vi "LowEnd-RT.vi"() -> ()   [LabVIEW 2016]
uses:
  <vilib>/rvi/interface/nirviOpenFPGA/nirviOpenFPGA.xnode
  <vilib>/rvi/interface/nirviReadWriteControl/nirviReadWriteControl.xnode
  LowEnd-FPGA.vi
  Controls/Glassman Control.ctl
  Controls/GP307 cluster.ctl
  Controls/Faraday cup states.ctl
  Controls/GV states.ctl
  Controls/Aperture states.ctl
  NiFpgaLv.dll
  <vilib>/Utility/error.llb/Error Cluster From Error Code.vi
  <vilib>/rvi/errors/niLvFpgaAdjustHostInterfaceError.vi
  <vilib>/NI_Real-Time Target Support.lvlib
  FPGA Bitfiles/PRIMEControl2017_FPGATarget2_LowEnd-FPGA_HC3RuQf6Dko.lvbitx
  <vilib>/FPGAPlugInAG/cRIO-9074/niLvFpga_Open_cRIO-9074.vi
panel:
  in  "Tab Control":T1(tab)
  out "LE Waist X+ Steerer V set":dbl
  out "LE Waist X+ Steerer HV Enable":bool
  out "LE Waist X- Steerer V set":dbl
  out "LE Waist X- Steerer HV Enable":bool
  out "LE Waist Y+ Steerer V set":dbl
  out "LE Waist Y+ Steerer HV Enable":bool
  out "LE Waist Y- Steerer V set":dbl
  out "LE Waist Y- Steerer HV Enable":bool
  out "LE Einzel V set":dbl
  out "LE Einzel HV Enable":bool
  out "LE Waist Y+ readback.V-monitor":fxp<+/-,16,5>
  out "LE Waist X+ readback.I-monitor":fxp<+/-,16,5>
  out "LE Waist X+ readback.V-monitor":fxp<+/-,16,5>
  out "LE Waist X- readback.I-monitor":fxp<+/-,16,5>
  out "LE Waist X- readback.V-monitor":fxp<+/-,16,5>
  out "LE Waist Y+ readback.I-monitor":fxp<+/-,16,5>
  out "LE Waist Y- readback.I-monitor":fxp<+/-,16,5>
  out "LE Waist Y- readback.V-monitor":fxp<+/-,16,5>
  out "LE Einzel readback.I-monitor":fxp<+/-,16,5>
  out "LE Einzel readback.V-monitor":fxp<+/-,16,5>
  out "Tank Entrance X+ Steerer HV Enable":bool
  out "Tank Entrance X+ Steerer V set":dbl
  out "Tank Entrance X- Steerer HV Enable":bool
  out "Tank Entrance X- Steerer V set":dbl
  out "Tank Entrance Y1+ Steerer HV Enable":bool
  out "Tank Entrance Y1+ Steerer V set":dbl
  out "Tank Entrance Y1- Steerer HV Enable":bool
  out "Tank Entrance Y1- Steerer V set":dbl
  out "Tank Entrance Y2+ Steerer HV Enable":bool
  out "Tank Entrance Y2+ Steerer V set":dbl
  out "Tank Entrance Y2- Steerer HV Enable":bool
  out "Tank Entrance Y2- Steerer V set":dbl
  out "Tank Entrance X+ readback.I-monitor":fxp<+/-,16,5>
  out "Tank Entrance X+ readback.V-monitor":fxp<+/-,16,5>
  out "Tank Entrance X- readback.I-monitor":fxp<+/-,16,5>
  out "Tank Entrance X- readback.V-monitor":fxp<+/-,16,5>
  out "Tank Entrance Y1+ readback.I-monitor":fxp<+/-,16,5>
  out "Tank Entrance Y1+ readback.V-monitor":fxp<+/-,16,5>
  out "Tank Entrance Y1- readback.I-monitor":fxp<+/-,16,5>
  out "Tank Entrance Y1- readback.V-monitor":fxp<+/-,16,5>
  out "Tank Entrance Y2+ readback.I-monitor":fxp<+/-,16,5>
  out "Tank Entrance Y2+ readback.V-monitor":fxp<+/-,16,5>
  out "Tank Entrance Y2- readback.I-monitor":fxp<+/-,16,5>
  out "Tank Entrance Y2- readback.V-monitor":fxp<+/-,16,5>
  out "LE Waist Vac Cluster":T2
  out "Tank Entrance Vac Cluster":T2
  out "LowEnd Waist Ion Gauge 1":u8[](array[numeric])
  out "LowEnd Waist Convectron 1":u8[](array[numeric])
  out "LowEnd Waist Ion Gauge 2":u8[](array[numeric])
  out "LowEnd Waist Convectron 2":u8[](array[numeric])
  out "LowEnd Waist Vac Interlock":bool
  out "Tank Entrance Vac Interlock":bool
  out "LowEnd Waist Vac Interlock bypass":bool
  out "Tank Entrance Vac Interlock bypass":bool
  out "Tank Entrance Ion Gauge 1":u8[](array[numeric])
  out "Tank Entrance Convectron 1":u8[](array[numeric])
  out "Tank Entrance Ion Gauge 2":u8[](array[numeric])
  out "Tank Entrance Convectron 2":u8[](array[numeric])
  out "Cryo Pump GV Position":T3
  out "Cryo Pump GV status":T4
  out "Beamline GV Position":T3
  out "Beamline GV status":T4
  out "Turbo GV Position":T3
  out "Turbo GV status":T4
  out "Tank Entrance FC Position":cluster{"IN sensor":bool, "OUT sensor":bool}
  out "Tank Entrance FC Status":T5
  out "LowEnd Waist FC Position":cluster{"IN sensor":bool, "OUT sensor":bool}
  out "LowEnd Waist FC Status":T5
  out "Bounce Mag Image  Aperture Position":cluster{"IN sensor":bool, "OUT sensor":bool}
  out "Bounce Mag Image  Aperture Position":T6
  out "Turbo GV actuator":bool
  out "Beamline GV actuator":bool
  out "Cryo Pump GV actuator":bool
  out "Tank Entrance FC actuator":bool
  out "LowEnd Waist FC actuator":bool
  out "Bounce Magnet Image Aperture actuator":bool
  out "Vac readback loop error":errorcluster
  out "HV control loop 2 error":errorcluster
  out "HV readback 2 loop error":errorcluster
  out "HV control 2 loop error":errorcluster
  out "Actuator-Sensor loop error":errorcluster
  out "HV readback 1 loop error":errorcluster
  out "GV Interlock loop error":errorcluster
  out "Error Handler":errorcluster
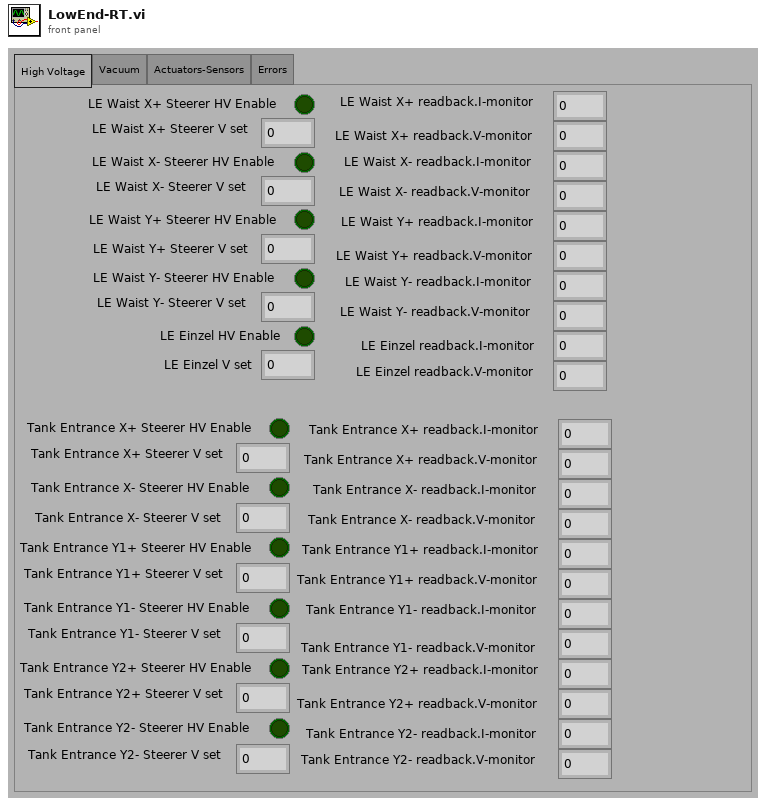
[diagram p1: front panel]
types:
  T1 = enum32{"High Voltage", "Vacuum", "Actuators-Sensors", "Errors"}
  T2 = cluster{"Ion gauge 1":string, "Convectron  Gauge 1 ":string, "Ion Gauge 2":string, "Convectrom Gauge 2":string}
  T3 = cluster{"OPEN sensor":bool, "Closed sensor":bool}
  T4 = typedef "GV states.ctl" = enum16{"status unclear", "closed", "open"}
  T5 = typedef "Faraday cup states.ctl" = enum16{"FC status unclear", "FC in", "FC out"}
  T6 = typedef "Aperture states.ctl" = enum16{"Aperture status unclear", "Aperture in", "Aperture out"}
  T7 = typedef "GP307 cluster.ctl" = cluster{"Ion gauge 1":string, "Convectron  Gauge 1 ":string, "Ion Gauge 2":string, "Convectrom Gauge 2":string}
  T8 = typedef "Glassman Control.ctl" = cluster{"V-program":fxp<+/-,16,5>, "HV Enable":bool}
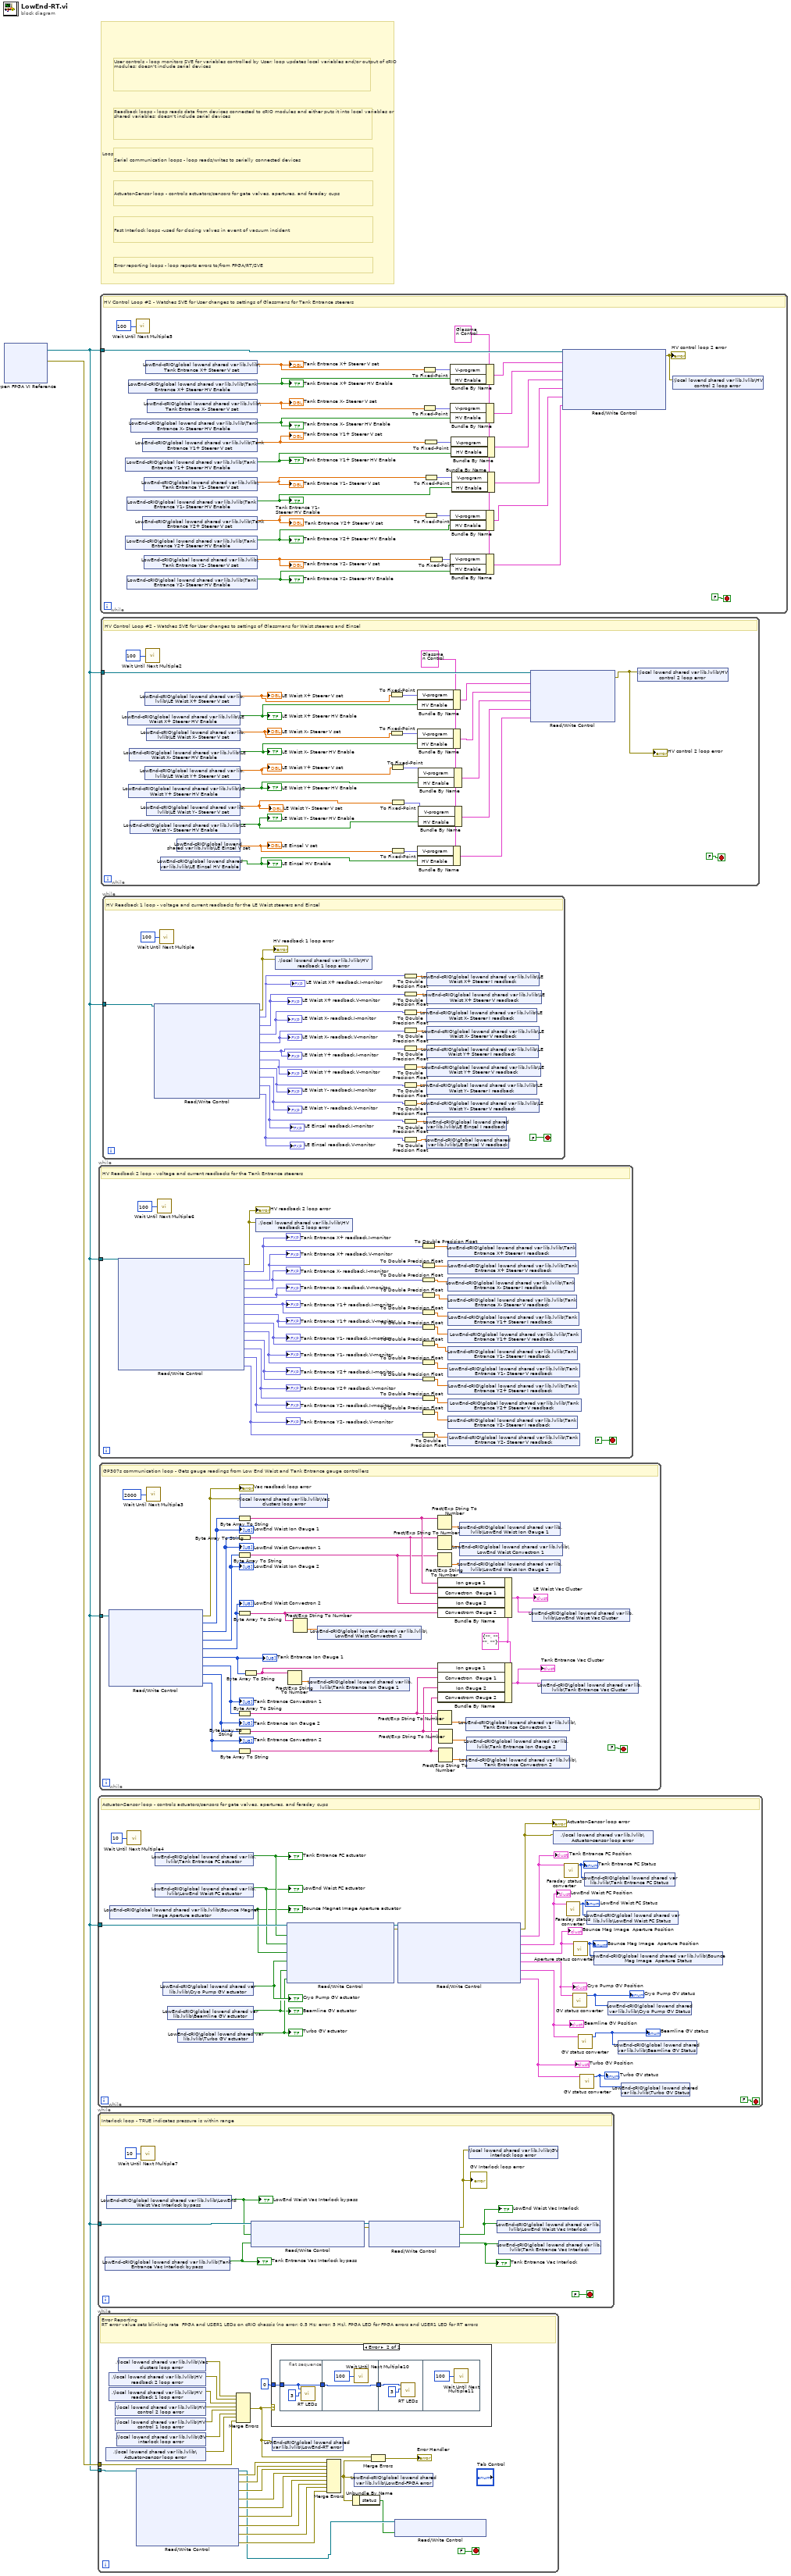
[diagram p0: block diagram]
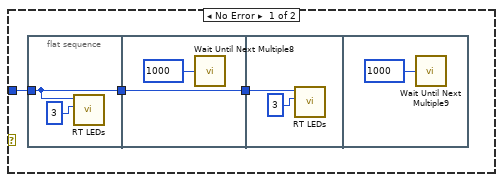
[diagram p2: hidden frame]
diagram:
  # "Actuator-Sensor loop - controls actuators/sensors for gate valves, apertures, and faraday cups"
  # "Fast Interlock loops -used for closing valves in event of vacuum incident"
  # "Error reporting loops - loop reports errors to/from FPGA/RT/SVE"
  # "Serial communication loops - loop reads/writes to serially connected devices"
  # "Readback loops - loop reads data from devices connected to cRIO modules and either puts it into local variables or shared variables; doesn't include serial devices"
  # "User controls - loop monitors SVE for variables controlled by User; loop updates local variables and/or output of cRIO modules; doesn't include serial devices"
  # "Loop legend - loops are color coded by responsibility"
  n1 = xnode "Open FPGA VI Reference"() -> ("FPGA VI Reference Out"=w1:refnum<k20>, "error out"=w2:errorcluster)  [unwired: 2 in]
  n2 = while {
    tunnel: w1 -> [w12]
    stop <- FALSE stop-if-true
    # "Interlock loop - TRUE indicates pressure is within range"
    n3 = shared-variable "LowEnd-cRIO\\global lowend shared var lib.lvlib\\Tank Entrance Vac Interlock bypass"() -> (w5:bool)  [unwired: 1 in, 1 out]
    "Tank Entrance Vac Interlock bypass" <- w5
    n4 = shared-variable "LowEnd-cRIO\\global lowend shared var lib.lvlib\\LowEnd Waist Vac Interlock bypass"() -> (w6:bool)  [unwired: 1 in, 1 out]
    "LowEnd Waist Vac Interlock bypass" <- w6
    n5 = call "Wait Until Next Multiple7"("Count(mSec)"=u32 10) -> ()  [unwired: 1 out]
    n6 = xnode "Read/Write Control"("FPGA VI Reference In"=w12, "LowEnd Waist Vac Interlock bypass"=w6, "Tank Entrance Vac Interlock bypass"=w5) -> ("FPGA VI Reference Out"=w11:refnum<k20>, "error out"=w10:errorcluster)  [unwired: 1 in]
    n7 = xnode "Read/Write Control"("FPGA VI Reference In"=w11, "error in"=w10) -> ("error out"=w9:errorcluster, "LowEnd Waist Vac Interlock"=w8:bool, "Tank Entrance Vac Interlock"=w7:bool)  [unwired: 1 out]
    "GV Interlock loop error" <- w9
    "LowEnd Waist Vac Interlock" <- w8
    "Tank Entrance Vac Interlock" <- w7
    n8 = shared-variable ".\\local lowend shared var lib.lvlib\\GV interlock loop error"(w9) -> ()  [unwired: 1 in, 1 out]
    n9 = shared-variable "LowEnd-cRIO\\global lowend shared var lib.lvlib\\LowEnd Waist Vac Interlock"(w8) -> ()  [unwired: 1 in, 1 out]
    n10 = shared-variable "LowEnd-cRIO\\global lowend shared var lib.lvlib\\Tank Entrance Vac Interlock"(w7) -> ()  [unwired: 1 in, 1 out]
  }
  n11 = while {
    tunnel: w1 -> [w36]
    tunnel: w2 -> [w16]
    stop <- FALSE stop-if-true
    # "Error Reporting\nRT error value sets blinking rate  FPGA and USER1 LEDs on cRIO chassis (no error: 0.5 Hz; error: 5 Hz). FPGA LED for FPGA errors and USER1 LED for RT errors"
    n12 = shared-variable ".\\local lowend shared var lib.lvlib\\Actuator-sensor loop error"() -> (w17:errorcluster)  [unwired: 1 in, 1 out]
    n13 = shared-variable ".\\local lowend shared var lib.lvlib\\HV readback 2 loop error"() -> (w22:errorcluster)  [unwired: 1 in, 1 out]
    n14 = shared-variable ".\\local lowend shared var lib.lvlib\\HV readback 1 loop error"() -> (w21:errorcluster)  [unwired: 1 in, 1 out]
    n15 = shared-variable ".\\local lowend shared var lib.lvlib\\HV control 2 loop error"() -> (w20:errorcluster)  [unwired: 1 in, 1 out]
    n16 = shared-variable ".\\local lowend shared var lib.lvlib\\HV control 1 loop error"() -> (w19:errorcluster)  [unwired: 1 in, 1 out]
    n17 = shared-variable ".\\local lowend shared var lib.lvlib\\GV interlock loop error"() -> (w18:errorcluster)  [unwired: 1 in, 1 out]
    n18 = shared-variable ".\\local lowend shared var lib.lvlib\\Vac clusters loop error"() -> (w23:errorcluster)  [unwired: 1 in, 1 out]
    n19 = xnode "Read/Write Control"("FPGA VI Reference In"=w36) -> ("FPGA VI Reference Out"=w25:refnum<k20>, "error out"=w26:errorcluster, "Low End Waist Vac Gauge error"=w27:errorcluster, "Tank Entrance Vac Gauge error"=w35:errorcluster, "GV Interlock loop error"=w34:errorcluster, "Actuator-sensor loop error"=w33:errorcluster, "HV control loop 1 error"=w32:errorcluster, "HV control loop 2 error"=w31:errorcluster, "HV readback loop #1 error"=w30:errorcluster, "HV readback loop #2 error"=w29:errorcluster)  [unwired: 1 in]
    n20 = Merge Errors(w23, w22, w21, w20, w19, w18, w17, w16) -> (w13:errorcluster)
    n21 = case shown="Error" w13 {
      tunnel: 0 -> [w40 w48]
      frame No Error {
        n22 = flat-sequence {
          tunnel: w40 -> [w41]
          tunnel: [w41] -> w38
          tunnel: [w43] -> w39
          tunnel: w38 -> [w43]
          tunnel: w39 -> [w45]
          frame #0 {
            n23 = call <vilib>:"RT LEDs.vi"("State"=3, "LED Num"=w41) -> ()  [unwired: 4 in, 2 out]
          }
          frame #1 {
            n24 = call "Wait Until Next Multiple8"("Count(mSec)"=u16 1000) -> ()  [unwired: 1 out]
          }
          frame #2 {
            n25 = call <vilib>:"RT LEDs.vi"("State"=3, "LED Num"=w45) -> ()  [unwired: 4 in, 2 out]
          }
          frame #3 {
            n26 = call "Wait Until Next Multiple9"("Count(mSec)"=u16 1000) -> ()  [unwired: 1 out]
          }
        }
      }
      frame Error {
        n27 = flat-sequence {
          tunnel: [w51] -> w50
          tunnel: w48 -> [w51]
          tunnel: w50 -> [w53]
          tunnel: [w53] -> w49
          tunnel: w49 -> [w55]
          frame #0 {
            n28 = call <vilib>:"RT LEDs.vi"("State"=3, "LED Num"=w51) -> ()  [unwired: 4 in, 2 out]
          }
          frame #1 {
            n29 = call "Wait Until Next Multiple10"("Count(mSec)"=u16 100) -> ()  [unwired: 1 out]
          }
          frame #2 {
            n30 = call <vilib>:"RT LEDs.vi"("State"=3, "LED Num"=w55) -> ()  [unwired: 4 in, 2 out]
          }
          frame #3 {
            n31 = call "Wait Until Next Multiple11"("Count(mSec)"=u16 100) -> ()  [unwired: 1 out]
          }
        }
      }
    }
    n32 = shared-variable "LowEnd-cRIO\\global lowend shared var lib.lvlib\\LowEnd-RT error"(w13) -> ()  [unwired: 1 in, 1 out]
    n33 = Merge Errors(w26, w27, w35, w34, w33, w32, w31, w30, w29) -> (w28:errorcluster)
    n34 = Unbundle By Name(w28) -> ("status"=w24:bool)
    n35 = shared-variable "LowEnd-cRIO\\global lowend shared var lib.lvlib\\LowEnd-FPGA error"(w28) -> ()  [unwired: 1 in, 1 out]
    n36 = Merge Errors(w13, w28) -> (→"Error Handler":errorcluster)
    n37 = xnode "Read/Write Control"("FPGA VI Reference In"=w25, "RT error"=w24) -> ()  [unwired: 1 in, 2 out]
  }
  n38 = while {
    tunnel: w1 -> [w81]
    stop <- FALSE stop-if-true
    # "Actuator-Sensor loop - controls actuators/sensors for gate valves, apertures, and faraday cups"
    n39 = shared-variable "LowEnd-cRIO\\global lowend shared var lib.lvlib\\Bounce Magnet Image Aperture actuator"() -> (w61:bool)  [unwired: 1 in, 1 out]
    "Bounce Magnet Image Aperture actuator" <- w61
    n40 = call "Wait Until Next Multiple4"("Count(mSec)"=u32 10) -> ()  [unwired: 1 out]
    n41 = shared-variable "LowEnd-cRIO\\global lowend shared var lib.lvlib\\LowEnd Waist FC actuator"() -> (w62:bool)  [unwired: 1 in, 1 out]
    "LowEnd Waist FC actuator" <- w62
    n42 = shared-variable "LowEnd-cRIO\\global lowend shared var lib.lvlib\\Tank Entrance FC actuator"() -> (w63:bool)  [unwired: 1 in, 1 out]
    "Tank Entrance FC actuator" <- w63
    n43 = shared-variable "LowEnd-cRIO\\global lowend shared var lib.lvlib\\Cryo Pump GV actuator"() -> (w60:bool)  [unwired: 1 in, 1 out]
    "Cryo Pump GV actuator" <- w60
    n44 = shared-variable "LowEnd-cRIO\\global lowend shared var lib.lvlib\\Beamline GV actuator"() -> (w58:bool)  [unwired: 1 in, 1 out]
    "Beamline GV actuator" <- w58
    n45 = shared-variable "LowEnd-cRIO\\global lowend shared var lib.lvlib\\Turbo GV actuator"() -> (w59:bool)  [unwired: 1 in, 1 out]
    "Turbo GV actuator" <- w59
    n46 = xnode "Read/Write Control"("FPGA VI Reference In"=w81, "Tank Entrance FC"=w63, "LowEnd Waist FC"=w62, "Bounce Magnet  Image Aperture"=w61, "Cryo Pump GV"=w60, "Beamline GV"=w58, "Turbo GV"=w59) -> ("FPGA VI Reference Out"=w79:refnum<k20>, "error out"=w77:errorcluster)  [unwired: 1 in]
    n47 = xnode "Read/Write Control"("FPGA VI Reference In"=w79, "error in"=w77) -> ("error out"=w64:errorcluster, "Tank Entrance FC Position"=w69:cluster{"IN sensor":bool, "OUT sensor":bool}, "LowEnd Waist FC Position"=w68:cluster{"IN sensor":bool, "OUT sensor":bool}, "Bounce Mag Image  Aperture Position"=w66:cluster{"IN sensor":bool, "OUT sensor":bool}, "Cryo Pump GV Position"=w75:T3, "Beamline GV Position"=w74:T3, "Turbo GV Position"=w73:T3)  [unwired: 1 out]
    "Cryo Pump GV Position" <- w75
    "Beamline GV Position" <- w74
    "Turbo GV Position" <- w73
    "Tank Entrance FC Position" <- w69
    "LowEnd Waist FC Position" <- w68
    "Bounce Mag Image  Aperture Position" <- w66
    "Actuator-Sensor loop error" <- w64
    n48 = shared-variable ".\\local lowend shared var lib.lvlib\\Actuator-sensor loop error"(w64) -> ()  [unwired: 1 in, 1 out]
    n49 = call "Faraday status converter.vi"("FC Position"=w69) -> ("FC Status"=w70:T5)  [unwired: 10 in]
    "Tank Entrance FC Status" <- w70
    n50 = call "Faraday status converter.vi"("FC Position"=w68) -> ("FC Status"=w67:T5)  [unwired: 10 in]
    "LowEnd Waist FC Status" <- w67
    n51 = call "GV status converter.vi"("Gate Valve"=w75) -> ("GV Status"=w71:T4)  [unwired: 10 in]
    "Cryo Pump GV status" <- w71
    n52 = call "Aperture status converter.vi"("Aperture Position"=w66) -> ("Aperture Status"=w65:T6)  [unwired: 10 in]
    "Bounce Mag Image  Aperture Position" <- w65
    n53 = call "GV status converter.vi"("Gate Valve"=w74) -> ("GV Status"=w76:T4)  [unwired: 10 in]
    "Beamline GV status" <- w76
    n54 = call "GV status converter.vi"("Gate Valve"=w73) -> ("GV Status"=w72:T4)  [unwired: 10 in]
    "Turbo GV status" <- w72
    n55 = shared-variable "LowEnd-cRIO\\global lowend shared var lib.lvlib\\Tank Entrance FC Status"(w70) -> ()  [unwired: 1 in, 1 out]
    n56 = shared-variable "LowEnd-cRIO\\global lowend shared var lib.lvlib\\LowEnd Waist FC Status"(w67) -> ()  [unwired: 1 in, 1 out]
    n57 = shared-variable "LowEnd-cRIO\\global lowend shared var lib.lvlib\\Bounce Mag Image  Aperture Status"(w65) -> ()  [unwired: 1 in, 1 out]
    n58 = shared-variable "LowEnd-cRIO\\global lowend shared var lib.lvlib\\Cryo Pump GV Status"(w71) -> ()  [unwired: 1 in, 1 out]
    n59 = shared-variable "LowEnd-cRIO\\global lowend shared var lib.lvlib\\Beamline GV Status"(w76) -> ()  [unwired: 1 in, 1 out]
    n60 = shared-variable "LowEnd-cRIO\\global lowend shared var lib.lvlib\\Turbo GV Status"(w72) -> ()  [unwired: 1 in, 1 out]
  }
  n61 = while {
    tunnel: w1 -> [w109]
    stop <- FALSE stop-if-true
    # "HV Readback 2 loop - voltage and current readbacks for the Tank Entrance steerers"
    n62 = xnode "Read/Write Control"("FPGA VI Reference In"=w109) -> ("error out"=w108:errorcluster, "Tank Entrance X+ readback.I-monitor"=w107:fxp<+/-,16,5>, "Tank Entrance X+ readback.V-monitor"=w106:fxp<+/-,16,5>, "Tank Entrance X- readback.I-monitor"=w105:fxp<+/-,16,5>, "Tank Entrance X- readback.V-monitor"=w104:fxp<+/-,16,5>, "Tank Entrance Y1+ readback.I-monitor"=w103:fxp<+/-,16,5>, "Tank Entrance Y1+ readback.V-monitor"=w102:fxp<+/-,16,5>, "Tank Entrance Y1- readback.I-monitor"=w101:fxp<+/-,16,5>, "Tank Entrance Y1- readback.V-monitor"=w100:fxp<+/-,16,5>, "Tank Entrance Y2+ readback.I-monitor"=w99:fxp<+/-,16,5>, "Tank Entrance Y2+ readback.V-monitor"=w98:fxp<+/-,16,5>, "Tank Entrance Y2- readback.I-monitor"=w97:fxp<+/-,16,5>, "Tank Entrance Y2- readback.V-monitor"=w96:fxp<+/-,16,5>)  [unwired: 1 in, 1 out]
    "HV readback 2 loop error" <- w108
    "Tank Entrance X+ readback.I-monitor" <- w107
    "Tank Entrance X+ readback.V-monitor" <- w106
    "Tank Entrance X- readback.I-monitor" <- w105
    "Tank Entrance X- readback.V-monitor" <- w104
    "Tank Entrance Y1+ readback.I-monitor" <- w103
    "Tank Entrance Y1+ readback.V-monitor" <- w102
    "Tank Entrance Y1- readback.I-monitor" <- w101
    "Tank Entrance Y1- readback.V-monitor" <- w100
    "Tank Entrance Y2+ readback.I-monitor" <- w99
    "Tank Entrance Y2+ readback.V-monitor" <- w98
    "Tank Entrance Y2- readback.I-monitor" <- w97
    "Tank Entrance Y2- readback.V-monitor" <- w96
    n63 = call "Wait Until Next Multiple6"("Count(mSec)"=u32 100) -> ()  [unwired: 1 out]
    n64 = shared-variable ".\\local lowend shared var lib.lvlib\\HV readback 2 loop error"(w108) -> ()  [unwired: 1 in, 1 out]
    n65 = To Double Precision Float(number=w107) -> (double precision float=w94:dbl)
    n66 = To Double Precision Float(number=w106) -> (double precision float=w93:dbl)
    n67 = To Double Precision Float(number=w105) -> (double precision float=w92:dbl)
    n68 = To Double Precision Float(number=w104) -> (double precision float=w91:dbl)
    n69 = To Double Precision Float(number=w103) -> (double precision float=w90:dbl)
    n70 = To Double Precision Float(number=w102) -> (double precision float=w89:dbl)
    n71 = To Double Precision Float(number=w101) -> (double precision float=w88:dbl)
    n72 = To Double Precision Float(number=w100) -> (double precision float=w87:dbl)
    n73 = To Double Precision Float(number=w99) -> (double precision float=w86:dbl)
    n74 = To Double Precision Float(number=w98) -> (double precision float=w85:dbl)
    n75 = To Double Precision Float(number=w97) -> (double precision float=w84:dbl)
    n76 = To Double Precision Float(number=w96) -> (double precision float=w83:dbl)
    n77 = shared-variable "LowEnd-cRIO\\global lowend shared var lib.lvlib\\Tank Entrance X+ Steerer I readback"(w94) -> ()  [unwired: 1 in, 1 out]
    n78 = shared-variable "LowEnd-cRIO\\global lowend shared var lib.lvlib\\Tank Entrance X+ Steerer V readback"(w93) -> ()  [unwired: 1 in, 1 out]
    n79 = shared-variable "LowEnd-cRIO\\global lowend shared var lib.lvlib\\Tank Entrance X- Steerer I readback"(w92) -> ()  [unwired: 1 in, 1 out]
    n80 = shared-variable "LowEnd-cRIO\\global lowend shared var lib.lvlib\\Tank Entrance X- Steerer V readback"(w91) -> ()  [unwired: 1 in, 1 out]
    n81 = shared-variable "LowEnd-cRIO\\global lowend shared var lib.lvlib\\Tank Entrance Y1+ Steerer I readback"(w90) -> ()  [unwired: 1 in, 1 out]
    n82 = shared-variable "LowEnd-cRIO\\global lowend shared var lib.lvlib\\Tank Entrance Y1+ Steerer V readback"(w89) -> ()  [unwired: 1 in, 1 out]
    n83 = shared-variable "LowEnd-cRIO\\global lowend shared var lib.lvlib\\Tank Entrance Y1- Steerer I readback"(w88) -> ()  [unwired: 1 in, 1 out]
    n84 = shared-variable "LowEnd-cRIO\\global lowend shared var lib.lvlib\\Tank Entrance Y1- Steerer V readback"(w87) -> ()  [unwired: 1 in, 1 out]
    n85 = shared-variable "LowEnd-cRIO\\global lowend shared var lib.lvlib\\Tank Entrance Y2+ Steerer I readback"(w86) -> ()  [unwired: 1 in, 1 out]
    n86 = shared-variable "LowEnd-cRIO\\global lowend shared var lib.lvlib\\Tank Entrance Y2+ Steerer V readback"(w85) -> ()  [unwired: 1 in, 1 out]
    n87 = shared-variable "LowEnd-cRIO\\global lowend shared var lib.lvlib\\Tank Entrance Y2- Steerer I readback"(w84) -> ()  [unwired: 1 in, 1 out]
    n88 = shared-variable "LowEnd-cRIO\\global lowend shared var lib.lvlib\\Tank Entrance Y2- Steerer V readback"(w83) -> ()  [unwired: 1 in, 1 out]
  }
  n89 = while {
    tunnel: w1 -> [w140]
    stop <- FALSE stop-if-true
    w122 = T7 {"Ion gauge 1"="", "Convectron  Gauge 1 "="", "Ion Gauge 2"="", "Convectrom Gauge 2"=""} ("Ion gauge cluster control")
    # "GP307s communication loop - Gets gauge readings from Low End Waist and Tank Entrance gauge controllers"
    n90 = xnode "Read/Write Control"("FPGA VI Reference In"=w140) -> ("error out"=w127:errorcluster, "Low End Waist Ion Gauge 1"=w139:u8[], "Low End Waist Convectron 1"=w138:u8[], "Low End Waist Ion Gauge 2"=w137:u8[], "Low End Waist Ion Gauge 2"=w136:u8[], "Tank Entrance Ion Gauge 1"=w126:u8[], "Tank Entrance Convectron 1"=w125:u8[], "Tank Entrance Ion Gauge 2"=w124:u8[], "Tank Entrance Convectron 2"=w123:u8[])  [unwired: 1 in, 1 out]
    "Vac readback loop error" <- w127
    "LowEnd Waist Ion Gauge 1" <- w139
    "LowEnd Waist Convectron 1" <- w138
    "LowEnd Waist Ion Gauge 2" <- w137
    "LowEnd Waist Convectron 2" <- w136
    "Tank Entrance Ion Gauge 1" <- w126
    "Tank Entrance Convectron 1" <- w125
    "Tank Entrance Ion Gauge 2" <- w124
    "Tank Entrance Convectron 2" <- w123
    n91 = call "Wait Until Next Multiple3"("Count(mSec)"=u32 2000) -> ()  [unwired: 1 out]
    n92 = Byte Array To String(unsigned byte array=w139) -> (string=w121:string)
    n93 = Byte Array To String(unsigned byte array=w138) -> (string=w120:string)
    n94 = Byte Array To String(unsigned byte array=w137) -> (string=w119:string)
    n95 = Byte Array To String(unsigned byte array=w136) -> (string=w118:string)
    n96 = Byte Array To String(unsigned byte array=w125) -> (string=w131:string)
    n97 = Byte Array To String(unsigned byte array=w124) -> (string=w130:string)
    n98 = Byte Array To String(unsigned byte array=w123) -> (string=w129:string)
    n99 = shared-variable ".\\local lowend shared var lib.lvlib\\Vac clusters loop error"(w127) -> ()  [unwired: 1 in, 1 out]
    n100 = Byte Array To String(unsigned byte array=w126) -> (string=w132:string)
    n101 = Fract/Exp String To Number(string=w132) -> (number=w112:dbl)  [unwired: 3 in, 1 out]
    n102 = Fract/Exp String To Number(string=w118) -> (number=w117:dbl)  [unwired: 3 in, 1 out]
    n103 = shared-variable "LowEnd-cRIO\\global lowend shared var lib.lvlib\\Tank Entrance Ion Gauge 1"(w112) -> ()  [unwired: 1 in, 1 out]
    n104 = shared-variable "LowEnd-cRIO\\global lowend shared var lib.lvlib\\LowEnd Waist Convectron 2"(w117) -> ()  [unwired: 1 in, 1 out]
    n105 = Fract/Exp String To Number(string=w121) -> (number=w114:dbl)  [unwired: 3 in, 1 out]
    n106 = Fract/Exp String To Number(string=w120) -> (number=w115:dbl)  [unwired: 3 in, 1 out]
    n107 = Fract/Exp String To Number(string=w119) -> (number=w116:dbl)  [unwired: 3 in, 1 out]
    n108 = Bundle By Name(cluster=w122, "Ion gauge 1"=w121, "Convectron  Gauge 1"=w120, "Ion Gauge 2"=w119, "Convectrom Gauge 2"=w118) -> (w133:T7)
    "LE Waist Vac Cluster" <- w133
    n109 = Bundle By Name(cluster=w122, "Ion gauge 1"=w132, "Convectron  Gauge 1"=w131, "Ion Gauge 2"=w130, "Convectrom Gauge 2"=w129) -> (w113:T7)
    "Tank Entrance Vac Cluster" <- w113
    n110 = Fract/Exp String To Number(string=w131) -> (number=w111:dbl)  [unwired: 3 in, 1 out]
    n111 = Fract/Exp String To Number(string=w130) -> (number=w110:dbl)  [unwired: 3 in, 1 out]
    n112 = Fract/Exp String To Number(string=w129) -> (number=w128:dbl)  [unwired: 3 in, 1 out]
    n113 = shared-variable "LowEnd-cRIO\\global lowend shared var lib.lvlib\\LowEnd Waist Convectron 1"(w115) -> ()  [unwired: 1 in, 1 out]
    n114 = shared-variable "LowEnd-cRIO\\global lowend shared var lib.lvlib\\LowEnd Waist Ion Gauge 1"(w114) -> ()  [unwired: 1 in, 1 out]
    n115 = shared-variable "LowEnd-cRIO\\global lowend shared var lib.lvlib\\LowEnd Waist Ion Gauge 2"(w116) -> ()  [unwired: 1 in, 1 out]
    n116 = shared-variable "LowEnd-cRIO\\global lowend shared var lib.lvlib\\Tank Entrance Convectron 1"(w111) -> ()  [unwired: 1 in, 1 out]
    n117 = shared-variable "LowEnd-cRIO\\global lowend shared var lib.lvlib\\Tank Entrance Ion Gauge 2"(w110) -> ()  [unwired: 1 in, 1 out]
    n118 = shared-variable "LowEnd-cRIO\\global lowend shared var lib.lvlib\\Tank Entrance Convectron 2"(w128) -> ()  [unwired: 1 in, 1 out]
    n119 = shared-variable "LowEnd-cRIO\\global lowend shared var lib.lvlib\\LowEnd Waist Vac Cluster"(w133) -> ()  [unwired: 1 in, 1 out]
    n120 = shared-variable "LowEnd-cRIO\\global lowend shared var lib.lvlib\\Tank Entrance Vac Cluster"(w113) -> ()  [unwired: 1 in, 1 out]
  }
  n121 = while {
    tunnel: w1 -> [w168]
    stop <- FALSE stop-if-true
    w148 = T8 {"V-program"=0.0, "HV Enable"=FALSE} ("Glassman Control")
    # "HV Control Loop #2 - Watches SVE for User changes to settings of Glassmans for Tank Entrance steerers"
    n122 = shared-variable "LowEnd-cRIO\\global lowend shared var lib.lvlib\\Tank Entrance Y1+ Steerer HV Enable"() -> (w156:bool)  [unwired: 1 in, 1 out]
    "Tank Entrance Y1+ Steerer HV Enable" <- w156
    n123 = shared-variable "LowEnd-cRIO\\global lowend shared var lib.lvlib\\Tank Entrance Y2+ Steerer HV Enable"() -> (w153:bool)  [unwired: 1 in, 1 out]
    "Tank Entrance Y2+ Steerer HV Enable" <- w153
    n124 = shared-variable "LowEnd-cRIO\\global lowend shared var lib.lvlib\\Tank Entrance Y1- Steerer HV Enable"() -> (w143:bool)  [unwired: 1 in, 1 out]
    "Tank Entrance Y1- Steerer HV Enable" <- w143
    n125 = shared-variable "LowEnd-cRIO\\global lowend shared var lib.lvlib\\Tank Entrance Y2- Steerer HV Enable"() -> (w151:bool)  [unwired: 1 in, 1 out]
    "Tank Entrance Y2- Steerer HV Enable" <- w151
    n126 = shared-variable "LowEnd-cRIO\\global lowend shared var lib.lvlib\\Tank Entrance X+ Steerer HV Enable"() -> (w160:bool)  [unwired: 1 in, 1 out]
    "Tank Entrance X+ Steerer HV Enable" <- w160
    n127 = shared-variable "LowEnd-cRIO\\global lowend shared var lib.lvlib\\Tank Entrance X- Steerer HV Enable"() -> (w158:bool)  [unwired: 1 in, 1 out]
    "Tank Entrance X- Steerer HV Enable" <- w158
    n128 = call "Wait Until Next Multiple5"("Count(mSec)"=u32 100) -> ()  [unwired: 1 out]
    n129 = shared-variable "LowEnd-cRIO\\global lowend shared var lib.lvlib\\Tank Entrance Y1+ Steerer V set"() -> (w157:dbl)  [unwired: 1 in, 1 out]
    "Tank Entrance Y1+ Steerer V set" <- w157
    n130 = shared-variable "LowEnd-cRIO\\global lowend shared var lib.lvlib\\Tank Entrance Y2+ Steerer V set"() -> (w154:dbl)  [unwired: 1 in, 1 out]
    "Tank Entrance Y2+ Steerer V set" <- w154
    n131 = shared-variable "LowEnd-cRIO\\global lowend shared var lib.lvlib\\Tank Entrance Y1- Steerer V set"() -> (w155:dbl)  [unwired: 1 in, 1 out]
    "Tank Entrance Y1- Steerer V set" <- w155
    n132 = shared-variable "LowEnd-cRIO\\global lowend shared var lib.lvlib\\Tank Entrance Y2- Steerer V set"() -> (w152:dbl)  [unwired: 1 in, 1 out]
    "Tank Entrance Y2- Steerer V set" <- w152
    n133 = shared-variable "LowEnd-cRIO\\global lowend shared var lib.lvlib\\Tank Entrance X+ Steerer V set"() -> (w161:dbl)  [unwired: 1 in, 1 out]
    "Tank Entrance X+ Steerer V set" <- w161
    n134 = shared-variable "LowEnd-cRIO\\global lowend shared var lib.lvlib\\Tank Entrance X- Steerer V set"() -> (w159:dbl)  [unwired: 1 in, 1 out]
    "Tank Entrance X- Steerer V set" <- w159
    n135 = To Fixed-Point(number=w161) -> (fixed-point=w167:fxp<+/-,16,5>)  [unwired: 1 in]
    n136 = To Fixed-Point(number=w159) -> (fixed-point=w166:fxp<+/-,16,5>)  [unwired: 1 in]
    n137 = To Fixed-Point(number=w157) -> (fixed-point=w165:fxp<+/-,16,5>)  [unwired: 1 in]
    n138 = To Fixed-Point(number=w155) -> (fixed-point=w164:fxp<+/-,16,5>)  [unwired: 1 in]
    n139 = To Fixed-Point(number=w154) -> (fixed-point=w163:fxp<+/-,16,5>)  [unwired: 1 in]
    n140 = To Fixed-Point(number=w152) -> (fixed-point=w162:fxp<+/-,16,5>)  [unwired: 1 in]
    n141 = Bundle By Name(cluster=w148, "V-program"=w167, "HV Enable"=w160) -> (w150:T8)
    n142 = Bundle By Name(cluster=w148, "V-program"=w166, "HV Enable"=w158) -> (w149:T8)
    n143 = Bundle By Name(cluster=w148, "V-program"=w163, "HV Enable"=w153) -> (w145:T8)
    n144 = Bundle By Name(cluster=w148, "V-program"=w162, "HV Enable"=w151) -> (w144:T8)
    n145 = Bundle By Name(cluster=w148, "V-program"=w165, "HV Enable"=w156) -> (w146:T8)
    n146 = Bundle By Name(cluster=w148, "V-program"=w164, "HV Enable"=w143) -> (w147:T8)
    n147 = xnode "Read/Write Control"("FPGA VI Reference In"=w168, "Tank Entrance X+ Steerer V set"=w150, "Tank Entrance X- Steerer V set"=w149, "Tank Entrance Y1+ Steerer V set"=w146, "Tank Entrance Y1- Steerer V set"=w147, "Tank Entrance Y2+ Steerer V set"=w145, "Tank Entrance Y2- Steerer V set"=w144) -> ("error out"=w142:errorcluster)  [unwired: 1 in, 1 out]
    "HV control loop 2 error" <- w142
    n148 = shared-variable ".\\local lowend shared var lib.lvlib\\HV control 2 loop error"(w142) -> ()  [unwired: 1 in, 1 out]
  }
  n149 = while {
    tunnel: w1 -> [w192]
    stop <- FALSE stop-if-true
    w186 = T8 {"V-program"=0.0, "HV Enable"=FALSE} ("Glassman Control")
    # "HV Control Loop #2 - Watches SVE for User changes to settings of Glassmans for Waist steerers and Einzel"
    n150 = shared-variable "LowEnd-cRIO\\global lowend shared var lib.lvlib\\LE Waist X+ Steerer HV Enable"() -> (w177:bool)  [unwired: 1 in, 1 out]
    "LE Waist X+ Steerer HV Enable" <- w177
    n151 = shared-variable "LowEnd-cRIO\\global lowend shared var lib.lvlib\\LE Waist Y+ Steerer HV Enable"() -> (w181:bool)  [unwired: 1 in, 1 out]
    "LE Waist Y+ Steerer HV Enable" <- w181
    n152 = shared-variable "LowEnd-cRIO\\global lowend shared var lib.lvlib\\LE Waist X- Steerer HV Enable"() -> (w179:bool)  [unwired: 1 in, 1 out]
    "LE Waist X- Steerer HV Enable" <- w179
    n153 = shared-variable "LowEnd-cRIO\\global lowend shared var lib.lvlib\\LE Waist Y- Steerer HV Enable"() -> (w184:bool)  [unwired: 1 in, 1 out]
    "LE Waist Y- Steerer HV Enable" <- w184
    n154 = shared-variable "LowEnd-cRIO\\global lowend shared var lib.lvlib\\LE Waist X+ Steerer V set"() -> (w176:dbl)  [unwired: 1 in, 1 out]
    "LE Waist X+ Steerer V set" <- w176
    n155 = shared-variable "LowEnd-cRIO\\global lowend shared var lib.lvlib\\LE Waist Y+ Steerer V set"() -> (w180:dbl)  [unwired: 1 in, 1 out]
    "LE Waist Y+ Steerer V set" <- w180
    n156 = call "Wait Until Next Multiple2"("Count(mSec)"=u32 100) -> ()  [unwired: 1 out]
    n157 = shared-variable "LowEnd-cRIO\\global lowend shared var lib.lvlib\\LE Waist X- Steerer V set"() -> (w178:dbl)  [unwired: 1 in, 1 out]
    "LE Waist X- Steerer V set" <- w178
    n158 = shared-variable "LowEnd-cRIO\\global lowend shared var lib.lvlib\\LE Waist Y- Steerer V set"() -> (w185:dbl)  [unwired: 1 in, 1 out]
    "LE Waist Y- Steerer V set" <- w185
    n159 = shared-variable "LowEnd-cRIO\\global lowend shared var lib.lvlib\\LE Einzel HV Enable"() -> (w182:bool)  [unwired: 1 in, 1 out]
    "LE Einzel HV Enable" <- w182
    n160 = shared-variable "LowEnd-cRIO\\global lowend shared var lib.lvlib\\LE Einzel V set"() -> (w183:dbl)  [unwired: 1 in, 1 out]
    "LE Einzel V set" <- w183
    n161 = To Fixed-Point(number=w176) -> (fixed-point=w191:fxp<+/-,16,5>)  [unwired: 1 in]
    n162 = To Fixed-Point(number=w178) -> (fixed-point=w190:fxp<+/-,16,5>)  [unwired: 1 in]
    n163 = To Fixed-Point(number=w180) -> (fixed-point=w189:fxp<+/-,16,5>)  [unwired: 1 in]
    n164 = To Fixed-Point(number=w185) -> (fixed-point=w188:fxp<+/-,16,5>)  [unwired: 1 in]
    n165 = To Fixed-Point(number=w183) -> (fixed-point=w187:fxp<+/-,16,5>)  [unwired: 1 in]
    n166 = Bundle By Name(cluster=w186, "V-program"=w191, "HV Enable"=w177) -> (w175:T8)
    n167 = Bundle By Name(cluster=w186, "V-program"=w190, "HV Enable"=w179) -> (w174:T8)
    n168 = Bundle By Name(cluster=w186, "V-program"=w187, "HV Enable"=w182) -> (w171:T8)
    n169 = Bundle By Name(cluster=w186, "V-program"=w189, "HV Enable"=w181) -> (w173:T8)
    n170 = Bundle By Name(cluster=w186, "V-program"=w188, "HV Enable"=w184) -> (w172:T8)
    n171 = xnode "Read/Write Control"("FPGA VI Reference In"=w192, "LE Waist X+ Steerer V set"=w175, "LE Waist X- Steerer V set"=w174, "LE Waist Y+ Steerer V set"=w173, "LE Waist Y- Steerer V set"=w172, "LE Einzel V set"=w171) -> ("error out"=w170:errorcluster)  [unwired: 1 in, 1 out]
    "HV control 2 loop error" <- w170
    n172 = shared-variable ".\\local lowend shared var lib.lvlib\\HV control 2 loop error"(w170) -> ()  [unwired: 1 in, 1 out]
  }
  n173 = while {
    tunnel: w1 -> [w217]
    stop <- FALSE stop-if-true
    # "HV Readback 1 loop - voltage and current readbacks for the LE Waist steerers and Einzel"
    n174 = xnode "Read/Write Control"("FPGA VI Reference In"=w217) -> ("error out"=w205:errorcluster, "LE Waist X+ readback.I-monitor"=w215:fxp<+/-,16,5>, "LE Waist X+ readback.V-monitor"=w206:fxp<+/-,16,5>, "LE Waist X- readback.I-monitor"=w207:fxp<+/-,16,5>, "LE Waist X- readback.V-monitor"=w208:fxp<+/-,16,5>, "LE Waist Y+ readback.I-monitor"=w209:fxp<+/-,16,5>, "LE Waist Y+ readback.V-monitor"=w210:fxp<+/-,16,5>, "LE Waist Y- readback.I-monitor"=w211:fxp<+/-,16,5>, "LE Waist Y- readback.V-monitor"=w212:fxp<+/-,16,5>, "LE Einzel readback.I-monitor"=w213:fxp<+/-,16,5>, "LE Einzel readback.V-monitor"=w214:fxp<+/-,16,5>)  [unwired: 1 in, 1 out]
    "HV readback 1 loop error" <- w205
    "LE Waist Y+ readback.V-monitor" <- w210
    "LE Waist X+ readback.I-monitor" <- w215
    "LE Waist X+ readback.V-monitor" <- w206
    "LE Waist X- readback.I-monitor" <- w207
    "LE Waist X- readback.V-monitor" <- w208
    "LE Waist Y+ readback.I-monitor" <- w209
    "LE Waist Y- readback.I-monitor" <- w211
    "LE Waist Y- readback.V-monitor" <- w212
    "LE Einzel readback.I-monitor" <- w213
    "LE Einzel readback.V-monitor" <- w214
    n175 = call "Wait Until Next Multiple"("Count(mSec)"=u32 100 ("millisecond multiple")) -> ()  [unwired: 1 out]
    n176 = shared-variable ".\\local lowend shared var lib.lvlib\\HV readback 1 loop error"(w205) -> ()  [unwired: 1 in, 1 out]
    n177 = To Double Precision Float(number=w215) -> (double precision float=w195:dbl)
    n178 = To Double Precision Float(number=w206) -> (double precision float=w196:dbl)
    n179 = To Double Precision Float(number=w207) -> (double precision float=w197:dbl)
    n180 = To Double Precision Float(number=w208) -> (double precision float=w198:dbl)
    n181 = To Double Precision Float(number=w209) -> (double precision float=w199:dbl)
    n182 = To Double Precision Float(number=w210) -> (double precision float=w200:dbl)
    n183 = To Double Precision Float(number=w211) -> (double precision float=w201:dbl)
    n184 = To Double Precision Float(number=w212) -> (double precision float=w202:dbl)
    n185 = To Double Precision Float(number=w213) -> (double precision float=w203:dbl)
    n186 = To Double Precision Float(number=w214) -> (double precision float=w204:dbl)
    n187 = shared-variable "LowEnd-cRIO\\global lowend shared var lib.lvlib\\LE Waist X+ Steerer I readback"(w195) -> ()  [unwired: 1 in, 1 out]
    n188 = shared-variable "LowEnd-cRIO\\global lowend shared var lib.lvlib\\LE Waist X+ Steerer V readback"(w196) -> ()  [unwired: 1 in, 1 out]
    n189 = shared-variable "LowEnd-cRIO\\global lowend shared var lib.lvlib\\LE Waist X- Steerer I readback"(w197) -> ()  [unwired: 1 in, 1 out]
    n190 = shared-variable "LowEnd-cRIO\\global lowend shared var lib.lvlib\\LE Waist X- Steerer V readback"(w198) -> ()  [unwired: 1 in, 1 out]
    n191 = shared-variable "LowEnd-cRIO\\global lowend shared var lib.lvlib\\LE Waist Y+ Steerer I readback"(w199) -> ()  [unwired: 1 in, 1 out]
    n192 = shared-variable "LowEnd-cRIO\\global lowend shared var lib.lvlib\\LE Waist Y+ Steerer V readback"(w200) -> ()  [unwired: 1 in, 1 out]
    n193 = shared-variable "LowEnd-cRIO\\global lowend shared var lib.lvlib\\LE Waist Y- Steerer I readback"(w201) -> ()  [unwired: 1 in, 1 out]
    n194 = shared-variable "LowEnd-cRIO\\global lowend shared var lib.lvlib\\LE Waist Y- Steerer V readback"(w202) -> ()  [unwired: 1 in, 1 out]
    n195 = shared-variable "LowEnd-cRIO\\global lowend shared var lib.lvlib\\LE Einzel I readback"(w203) -> ()  [unwired: 1 in, 1 out]
    n196 = shared-variable "LowEnd-cRIO\\global lowend shared var lib.lvlib\\LE Einzel V readback"(w204) -> ()  [unwired: 1 in, 1 out]
  }
